vi "Stop Core.vi"(10 "final error code":i32, 11 "DataLogger in":refnum<class "DataLogger.lvclass">) -> (3 "DataLogger out":refnum<class "DataLogger.lvclass">)   [LabVIEW 2019, in "DataLogger.lvclass"]
doc: "(<B>Filename</B>: Actor Framework.lvlib:Actor.lvclass:Stop Core.vi)\n\nDefines what the actor does before it stops. Use the <B>final error code</B> input to determine whether the actor shut down in response to an error.\n\nBy default, this method does nothing. A descendant class may override it to define behavior, such as shutting down any processes the actor initiated in its override of the Actor Core method."
uses:
  DataLogger.lvclass
  <vilib>/ActorFramework/Actor/Actor.lvclass
panel:
  out "error out":errorcluster
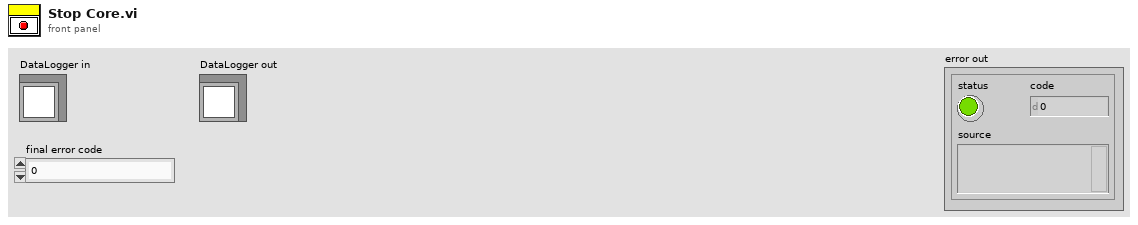
[diagram p1: front panel]
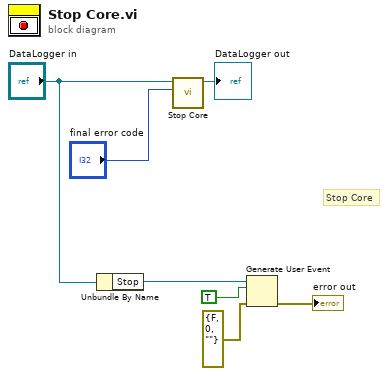
[diagram p0: block diagram]
diagram:
  # "Stop Core"
  n1 = Unbundle By Name("DataLogger in") -> ("Stop"=w4:refnum<user-event>)
  n2 = call-parent "Stop Core.vi"("final error code"="final error code", "Actor in"="DataLogger in") -> ("Actor out"=→"DataLogger out":refnum<class "DataLogger.lvclass">)  [unwired: 9 in]
  n3 = Generate User Event(user event=w4, event data cluster=TRUE ("event data"), error in=errorcluster {"status"=FALSE, "code"=0, "source"=""} ("error in (no error)")) -> (error out=→"error out":errorcluster)  [unwired: 1 in, 1 out]
